vi "CC CryoCooler Data buffer.vi"(8 "error in (no error)":errorcluster, 9 "Write?":bool, 10 "Data":dbl[](array[numeric]), 11 "Time Stamp":timestamp) -> (0 "error out":errorcluster, 3 "XY Graph":T1(graph))   [LabVIEW 2021]
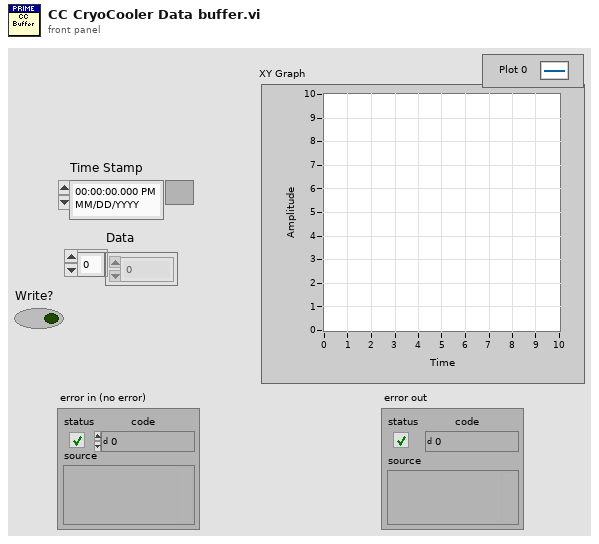
[diagram p1: front panel]
types:
  T1 = cluster{cluster{"Time Stamp":timestamp, "Numeric":dbl}[]}[]
  T2 = cluster{cluster{"Time Stamp":timestamp, "Numeric":dbl}[]}
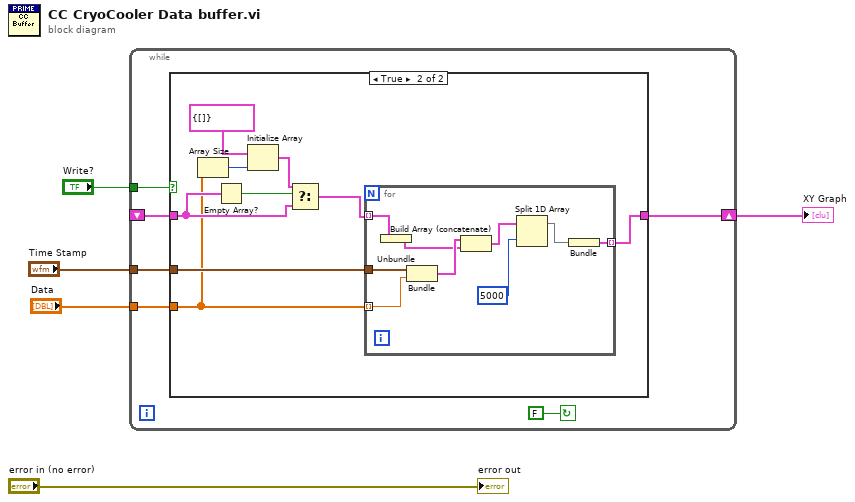
[diagram p0: block diagram]
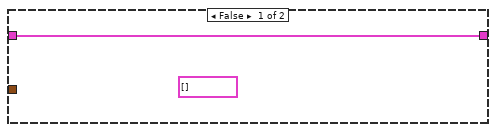
[diagram p2: hidden frame]
diagram:
  n1 = while {
    shift-right: [w7] -> w2
    shift-left: _ -> [w8]
    tunnel: "Data" -> [w10]
    tunnel: "Time Stamp" -> [w9]
    tunnel: "Write?" -> [w6]
    stop <- FALSE continue-if-true
    n2 = case shown="True" w6 {
      tunnel: w10 -> [_ w16]
      tunnel: w9 -> [_ w21]
      tunnel: w8 -> [w12 w18]
      tunnel: [w12 w20] -> w7
      frame False {
        (unwired) T1 []
      }
      frame True {
        n3 = Array Size(array=w16) -> (size(s)=w15:i32)
        n4 = Empty Array?(array=w18) -> (empty?=w19:bool)
        n5 = Initialize Array(T2 {[]}, w15) -> (w13:T1)
        n6 = Select(t=w13, s=w19, f=w18) -> (s? t:f=w17:T1)
        n7 = for {
          tunnel: w17 -> [w30] mode=indexing
          tunnel: w21 -> [w29]
          tunnel: w16 -> [w28] mode=indexing
          tunnel: [w25] -> w20 mode=indexing
          n8 = Unbundle(w30) -> (w26:cluster{"Time Stamp":timestamp, "Numeric":dbl}[])
          n9 = Bundle("Time Stamp"=w29, "Numeric"=w28) -> (w27:cluster{"Time Stamp":timestamp, "Numeric":dbl})  [unwired: 1 in]
          n10 = Build Array (concatenate)(w27, w26) -> (w24:cluster{"Time Stamp":timestamp, "Numeric":dbl}[])
          n11 = Split 1D Array(array=w24, index=5000) -> (first subarray=w22:cluster{"Time Stamp":timestamp, "Numeric":dbl}[])  [unwired: 1 out]
          n12 = Bundle(w22) -> (w25:T2)  [unwired: 1 in]
        }
      }
    }
  }
  "XY Graph" <- w2
  "error out" <- "error in (no error)"
